vi "VarreduraFreq.vi"() -> ()   [LabVIEW 2018]
uses:
  <vilib>/Analysis/baseanly.llb/Mean (DBL).vi
  <vilib>/Analysis/2dsp.llb/1D Convolution (DBL).vi
  <vilib>/Analysis/baseanly.llb/Mean (CDB).vi
  <vilib>/measure/maspectr.llb/FFT Power Spectrum and PSD for 1 Chan (CDB).vi
  <vilib>/Analysis/3filter.llb/Butterworth Filter (DBL).vi
  <vilib>/measure/maspectr.llb/FFT Power Spectrum and PSD for 1 Chan.vi
  <vilib>/measure/mamon.llb/Trigger Detection for 1 Channel.vi
  <vilib>/rtlsdr/rtlsdr.lvlib
  <vilib>/measure/NI_MAPro.lvlib
  <vilib>/Analysis/NI_AALBase.lvlib
  <vilib>/Analysis/NI_AALPro.lvlib
panel:
  in  "VBW (kHz)":dbl=0.12500000000000006 format="%0.4f"
  out "Histerese":dbl
  out "f0 (kHz)":dbl
  in  "RBW (kHz)":i32=9
  in  "Modulo":dbl
  in  "Exponêncial":dbl
  out "Decidas":dbl[](array[numeric])
  out "Subidas":dbl[](array[numeric])
  out "Limiar":dbl format="%0.2f"
  out "F Count":i32
  out "size(s)":i32
  out "Power Spectrum 2":cluster{"f0":dbl, "df":dbl, "magnitude":dbl[]}(graph)
  out "Power Spectrum":cluster{"f0":dbl, "df":dbl, "magnitude":dbl[]}[](graph)
  out "Center Frequency":dbl
  in  "config":bool
  in  "Number Of Samples":i32=16000
  in  "Center Frequency":u32=101000000
  in  "Sample Rate":u32=2400000
  out "function return":i32
  in  "Device Index":u32=1
  out "Device USB Strings":T1
  out "DeviceRefnum Out":u64
  in  "stop":bool
  out "Device Count":u32
  # "1"
  # "1,433"
  # "12,801"
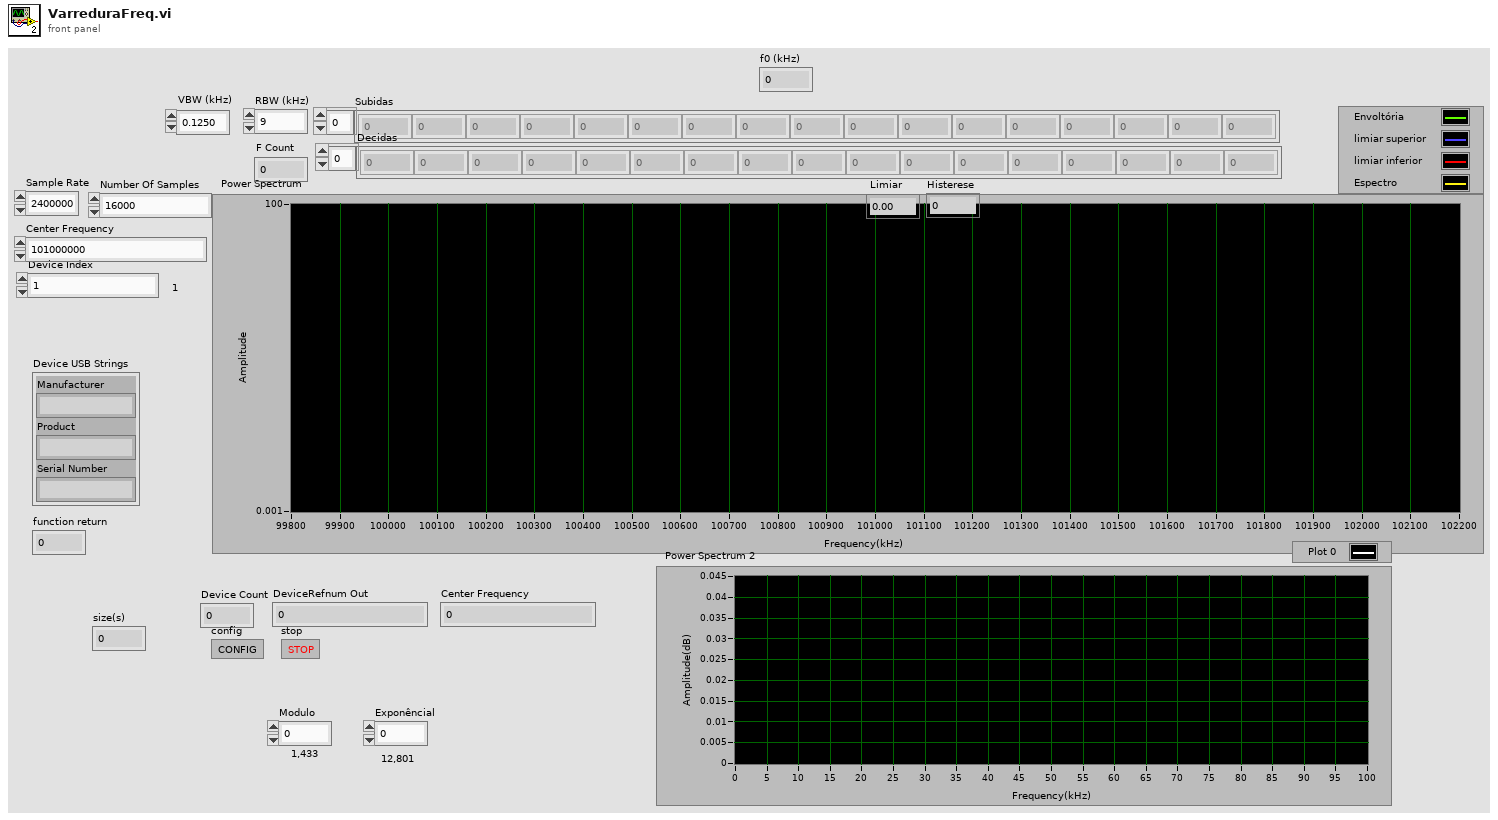
[diagram p1: front panel]
types:
  T1 = cluster{"Manufacturer":string, "Product":string, "Serial Number":string}
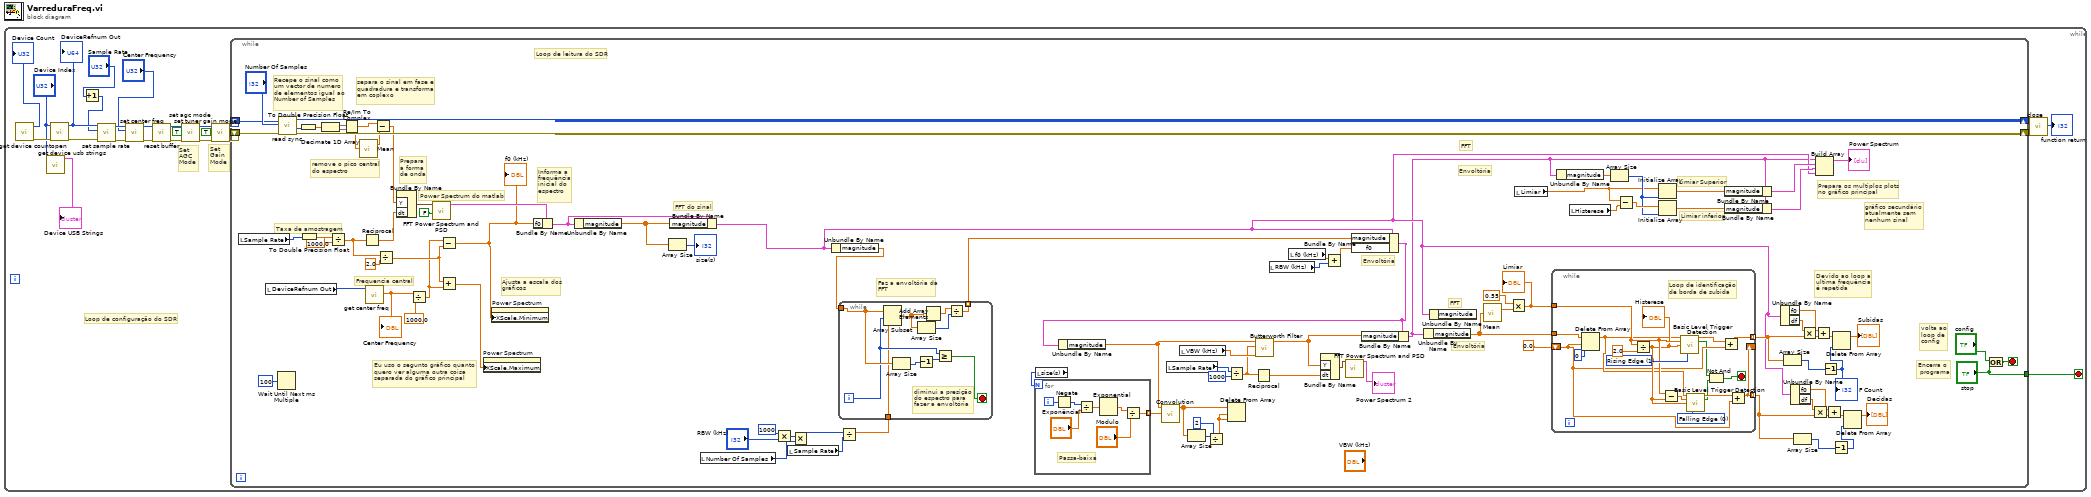
[diagram p0: block diagram]
diagram:
  n1 = while {
    stop <- w5 stop-if-true
    # "Set\nGain\nMode"
    # "Set\nAGC\nMode"
    # "Loop de configuração do SDR"
    n2 = call <vilib>:"get device count.vi"() -> ("error out"=w24:errorcluster, "Device Count"=→"Device Count":u32)  [unwired: 10 in]
    n3 = call <vilib>:"get device usb strings.vi"("Device Index"="Device Index") -> ("Device USB Strings"=→"Device USB Strings":T1)  [unwired: 8 in, 2 out]
    n4 = call <vilib>:"open.vi"("error in (no error)"=w24, "Device Index"="Device Index") -> ("error out"=w20:errorcluster, "DeviceRefnum Out"=w19:u64)  [unwired: 6 in]
    "DeviceRefnum Out" <- w19
    n5 = Increment(x="Sample Rate") -> (x+1=w1:u32)
    n6 = call <vilib>:"set sample rate.vi"("error in (no error)"=w20, "Sample Rate"=w1, "DeviceRefnum"=w19) -> ("error out"=w18:errorcluster, "DeviceRefnum Out"=w17:u64)  [unwired: 6 in, 1 out]
    n7 = call <vilib>:"set center freq.vi"("error in (no error)"=w18, "Center Frequency"="Center Frequency", "DeviceRefnum"=w17) -> ("error out"=w16:errorcluster, "DeviceRefnum Out"=w15:u64)  [unwired: 6 in, 1 out]
    n8 = call <vilib>:"reset buffer.vi"("error in (no error)"=w16, "DeviceRefnum"=w15) -> ("error out"=w14:errorcluster, "DeviceRefnum Out"=w13:u64)  [unwired: 7 in, 1 out]
    n9 = call <vilib>:"set agc mode.vi"("error in (no error)"=w14, "AGC Enable"=TRUE, "DeviceRefnum"=w13) -> ("error out"=w12:errorcluster, "DeviceRefnum Out"=w11:u64)  [unwired: 6 in, 1 out]
    n10 = call <vilib>:"set tuner gain mode.vi"("error in (no error)"=w12, "AutoGain"=TRUE ("AGC Enable"), "DeviceRefnum"=w11) -> ("error out"=w9:errorcluster, "DeviceRefnum Out"=w8:u64)  [unwired: 6 in, 1 out]
    n11 = while {
      shift-right: [w107] -> w6
      shift-left: w8 -> [w96]
      shift-right: [w108] -> w7
      shift-left: w9 -> [w109]
      tunnel: ["stop"] -> w5
      stop <- w120 stop-if-true
      # "gráfico secundário\natualmente sem \nnenhum sinal"
      # "Prepara os multiplos plots\nno gráfico principal"
      # "Limiar inferior"
      # "Limiar Superior"
      # "FFT"
      # "Envoltória"
      # "Informa a \nfrequência\ninicial do\nespectro"
      # "Prepara \na forma \nde onda"
      # "Taxa de amostragem"
      # "Frequencia central"
      # "Eu uso o segunto gráfico quanto \nquero ver alguma outra coisa \nseparada do gráfico principal"
      # "Devido ao loop a\nultima frequência\né repetida"
      # "FFT"
      # "Envoltória"
      # "Envoltória"
      # "Faz a envoltória da\nFFT"
      # "FFT do sinal"
      # "remove o pico central\ndo espectro"
      # "Ajusta a escala dos\ngráficos"
      # "separa o sinal em fase e\nquadradura e transforma\nem coplexo"
      # "Recepe o sinal como\num vector de numero\nde elementos igual ao\nNumber of Samples"
      # "Encerra o\n programa"
      # "volta ao\nloop de \nconfig"
      # "Power Spectrum do matlab"
      # "Loop de leitura do SDR"
      n12 = local read "Sample Rate"() -> (w44:u32)
      n13 = local read "DeviceRefnum Out"() -> (w63:u64)
      n14 = Wait Until Next ms Multiple(millisecond multiple=u32 100) -> ()  [unwired: 1 out]
      n15 = call <vilib>:"read sync.vi"("error in (no error)"=w109, "Number Of Samples"="Number Of Samples", "DeviceRefnum"=w96) -> ("error out"=w108:errorcluster, "Sample Buffer"=w106:u8[], "DeviceRefnum Out"=w107:u64)  [unwired: 5 in, 1 out]
      n16 = To Double Precision Float(number=w106) -> (double precision float=w103:dbl[])
      n17 = To Double Precision Float(number=w44) -> (double precision float=w111:dbl)
      n18 = Decimate 1D Array(w103) -> (w104:dbl[], w105:dbl[])
      n19 = Divide(x=w111, y=1000.0) -> (x/y=w114:dbl)
      n20 = Re/Im To Complex(1:w105, 2:w104) -> (0:w62:cdb[])
      n21 = call-poly <vilib>:"Mean.vi"("X"=w62) -> ("mean"=w61:cdb)  [unwired: 1 out]
      n22 = Reciprocal(x=w114) -> (1/x=w102:dbl)
      n23 = call <vilib>:"get center freq.vi"("DeviceRefnum"=w63) -> ("Center Frequency"=w95:dbl)  [unwired: 8 in, 2 out]
      "Center Frequency" <- w95
      n24 = Subtract(x=w62, y=w61) -> (x-y=w39:cdb[])
      n25 = Divide(x=w114, y=2.0) -> (x/y=w100:dbl)
      n26 = Bundle By Name("Y"=w39, "dt"=w102) -> (w116:waveform(cdb))  [unwired: 1 in]
      n27 = Divide(x=w95, y=1000.0) -> (x/y=w99:dbl)
      n28 = call-poly <vilib>:"FFT Power Spectrum and PSD.vi"("dB On (F)"=FALSE, "time signal"=w116) -> ("Power Spectrum / PSD"=w101:cluster{"f0":dbl, "df":dbl, "magnitude":dbl[]})  [unwired: 6 in, 3 out]
      n29 = Subtract(x=w99, y=w100) -> (x-y=w98:dbl)
      "f0 (kHz)" <- w98
      n30 = Add(x=w100, y=w99) -> (x+y=w110:dbl)
      n31 = property on="Power Spectrum" class="WFGraph (strict)"("XScale.Maximum"=w110) -> ()  [unwired: 2 in, 2 out]
      n32 = property on="Power Spectrum" class="WFGraph (strict)"("XScale.Minimum"=w98) -> ()  [unwired: 2 in, 2 out]
      n33 = Bundle By Name(cluster=w101, "f0"=w98) -> (w93:cluster{"f0":dbl, "df":dbl, "magnitude":dbl[]})
      n34 = Unbundle By Name(w93) -> ("magnitude"=w94:dbl[])
      n35 = Array Size(array=w94) -> (size(s)=→"size(s)":i32)
      n36 = Bundle By Name(cluster=w93, "magnitude"=w94) -> (w37:cluster{"f0":dbl, "df":dbl, "magnitude":dbl[]})
      n37 = local read "Number Of Samples"() -> (w49:i32)
      n38 = Multiply(x=1000, y="RBW (kHz)") -> (x*y=w52:i32)
      n39 = local read "Sample Rate"() -> (w47:u32)
      n40 = Multiply(x=w52, y=w49) -> (x*y=w50:i32)
      n41 = Unbundle By Name(w37) -> ("magnitude"=w40:dbl[])
      n42 = Divide(x=w50, y=w47) -> (x/y=w48:dbl)
      n43 = while {
        tunnel: w40 -> [w137]
        tunnel: w48 -> [w130]
        tunnel: [w129] -> w41 mode=indexing
        i -> [w136]
        stop <- w135 stop-if-true
        # "diminui a presição \ndo espectro para \nfazer a envoltória"
        n44 = Array Subset(array=w137, index=w136, length=w130) -> (w133:dbl[])
        n45 = Array Size(array=w137) -> (size(s)=w132:i32)
        n46 = Decrement(x=w132) -> (x-1=w131:i32)
        n47 = Array Size(array=w133) -> (size(s)=w134:i32)
        n48 = Add Array Elements(numeric array=w133) -> (sum=w138:dbl)
        n49 = Greater Or Equal?(x=w136, y=w131) -> (x >= y?=w135:bool)
        n50 = Divide(x=w138, y=w134) -> (x/y=w129:dbl)
      }
      n51 = local read "size(s)"() -> (w60:i32)
      n52 = for {
        N: w60 -> [_]
        tunnel: [w122] -> w59 mode=indexing
        i -> [w128]
        # "Passa-baixa"
        n53 = Negate(x=w128) -> (-x=w127:i32)
        n54 = Divide(x=w127, y="Exponêncial") -> (x/y=w125:dbl)
        n55 = Exponential(1:w125) -> (0:w124:dbl)
        n56 = Divide(x=w124, y="Modulo") -> (x/y=w122:dbl)
      }
      n57 = local read "Sample Rate"() -> (w32:u32)
      n58 = local read "VBW (kHz)"() -> (w29:dbl)
      n59 = Divide(x=w32, y=u32 1000) -> (x/y=w28:dbl)
      n60 = Reciprocal(x=w28) -> (1/x=w30:dbl)
      n61 = local read "RBW (kHz)"() -> (w45:i32)
      n62 = local read "f0 (kHz)"() -> (w46:dbl)
      n63 = Add(x=w46, y=w45) -> (x+y=w35:dbl)
      n64 = Bundle By Name(cluster=w37, "magnitude"=w41, "f0"=w35) -> (w33:cluster{"f0":dbl, "df":dbl, "magnitude":dbl[]})
      n65 = Unbundle By Name(w33) -> ("magnitude"=w27:dbl[])
      n66 = call-poly <vilib>:"Convolution.vi"("Y"=w59, "X"=w27) -> ("X * Y"=w55:dbl[])  [unwired: 8 in, 1 out]
      n67 = Array Size(array=w55) -> (size(s)=w58:i32)
      n68 = Divide(x=w58, y=2) -> (x/y=w56:dbl)
      n69 = Delete From Array(array=w55, length=w56, index=w56) -> ()  [unwired: 2 out]
      n70 = call-poly <vilib>:"Butterworth Filter.vi"("low cutoff freq: fl"=w29, "sampling freq: fs"=w28, "X"=w27) -> ("Filtered X"=w26:dbl[])  [unwired: 5 in, 1 out]
      n71 = Bundle By Name("Y"=w26, "dt"=w30) -> (w38:waveform(dbl))  [unwired: 1 in]
      n72 = call-poly <vilib>:"FFT Power Spectrum and PSD.vi"("time signal"=w38) -> ("Power Spectrum / PSD"=→"Power Spectrum 2":cluster{"f0":dbl, "df":dbl, "magnitude":dbl[]})  [unwired: 7 in, 3 out]
      n73 = Bundle By Name(cluster=w33, "magnitude"=w26) -> (w34:cluster{"f0":dbl, "df":dbl, "magnitude":dbl[]})
      n74 = Unbundle By Name(w34) -> ("magnitude"=w54:dbl[])
      n75 = Unbundle By Name(w37) -> ()  [unwired: 1 out]
      n76 = call-poly <vilib>:"Mean.vi"("X"=w54) -> ("mean"=w90:dbl)  [unwired: 1 out]
      n77 = Multiply(x=0.55, y=w90) -> (x*y=w84:dbl)
      "Limiar" <- w84
      n78 = local read "Limiar"() -> (w43:dbl)
      n79 = while {
        tunnel: [w151] -> w87 mode=indexing
        shift-right: [w141] -> _
        shift-left: 0.0 -> [w142]
        tunnel: w54 -> [w148]
        tunnel: w84 -> [w146]
        tunnel: [w141] -> w67 mode=indexing
        stop <- w154 stop-if-true
        w149 = u16 0 items=["Falling Edge", "Rising Edge"] ("trigger slope")
        w155 = u16 1 items=["Falling Edge", "Rising Edge"] ("trigger slope")
        # "Loop de identificação\nde borda de subida"
        n80 = Delete From Array(array=w148, length=w142, index=0) -> (array with subset deleted=w143:dbl[])  [unwired: 1 out]
        n81 = Divide(x=w146, y=2.0) -> (x/y=w145:dbl)
        "Histerese" <- w145
        n82 = Subtract(x=w146, y=w145) -> (x-y=w147:dbl)
        n83 = call-poly <vilib>:"Basic Level Trigger Detection.vi"("signal in"=w143, "level"=w146, "hysteresis"=w145, "trigger slope"=w155) -> ("trigger location"=w152:dbl, "trigger detected?"=w140:bool)  [unwired: 9 in, 1 out]
        n84 = call-poly <vilib>:"Basic Level Trigger Detection.vi"("signal in"=w143, "level"=w147, "hysteresis"=w145, "trigger slope"=w149) -> ("trigger location"=w144:dbl, "trigger detected?"=w139:bool)  [unwired: 9 in, 1 out]
        n85 = Not And(1:w139, 2:w140) -> (0:w154:bool)
        n86 = Add(x=w152, y=w142) -> (x+y=w151:dbl)
        n87 = Add(x=w144, y=w142) -> (x+y=w141:dbl)
      }
      n88 = Unbundle By Name(w34) -> ("magnitude"=w83:dbl[])
      n89 = local read "Histerese"() -> (w42:dbl)
      n90 = Array Size(array=w83) -> (size(s)=w82:i32)
      n91 = Subtract(x=w43, y=w42) -> (x-y=w85:dbl)
      n92 = Initialize Array(w43, w82) -> (w80:dbl[])
      n93 = Initialize Array(w85, w82) -> (w81:dbl[])
      n94 = Bundle By Name(cluster=w34, "magnitude"=w80) -> (w64:cluster{"f0":dbl, "df":dbl, "magnitude":dbl[]})
      n95 = Bundle By Name(cluster=w34, "magnitude"=w81) -> (w65:cluster{"f0":dbl, "df":dbl, "magnitude":dbl[]})
      n96 = Unbundle By Name(w37) -> ("f0"=w74:dbl, "df"=w76:dbl)
      n97 = Array Size(array=w87) -> (size(s)=w86:i32)
      n98 = Unbundle By Name(w37) -> ("f0"=w68:dbl, "df"=w70:dbl)
      n99 = Array Size(array=w67) -> (size(s)=w73:i32)
      n100 = Multiply(x=w76, y=w87) -> (x*y=w77:dbl[])
      n101 = Multiply(x=w70, y=w67) -> (x*y=w71:dbl[])
      n102 = Add(x=w74, y=w77) -> (x+y=w75:dbl[])
      n103 = Build Array(w34, w64, w65, w37) -> (→"Power Spectrum":cluster{"f0":dbl, "df":dbl, "magnitude":dbl[]}[])
      n104 = Decrement(x=w86) -> (x-1=w78:i32)
      "F Count" <- w78
      n105 = Add(x=w68, y=w71) -> (x+y=w69:dbl[])
      n106 = Decrement(x=w73) -> (x-1=w72:i32)
      n107 = Delete From Array(array=w75, index=w78) -> (array with subset deleted=→"Subidas":dbl[])  [unwired: 1 in, 1 out]
      n108 = Delete From Array(array=w69, index=w72) -> (array with subset deleted=→"Decidas":dbl[])  [unwired: 1 in, 1 out]
      n109 = Or(x="config", y="stop") -> (x .or. y?=w120:bool)
    }
    n110 = call <vilib>:"close.vi"("error in (no error)"=w7, "DeviceRefnum"=w6) -> ("function return"=→"function return":i32)  [unwired: 8 in, 1 out]
  }
